vi "Basic Multitone with Amplitudes.vi"(0 "start frequency":dbl=10.0 format="%0.2f", 2 "reset signal":bool, 3 "amplitude":dbl=-1.0 format="%0.2f", 5 "tone amplitudes":dbl[](array[numeric])=[1.0, 2.0] format="%0.2f", 7 "seed":i32=-1, 9 "delta frequency":dbl=100.0 format="%0.2f", 11 "error in (no error)":errorcluster, 12 "sampling info":cluster{"Fs":dbl, "#s":dbl}={"Fs"=1000.0, "#s"=1000.0} {"Fs" format="%.1p"}, 13 "coerce frequencies?":bool, 14 "phase relationship":u16(ring) items=["random", "linear difference", "linear phase"]) -> (4 "signal out":waveform(dbl), 6 "crest factor":dbl format="%0.2f", 10 "actual tone frequencies":dbl[](array[numeric]), 15 "error out":errorcluster)   [LabVIEW 2020, in "NI_MAPro.lvlib"]
doc: "Generates a waveform that is the sum of integer cycle sine tones."
uses:
  NI_MAPro.lvlib
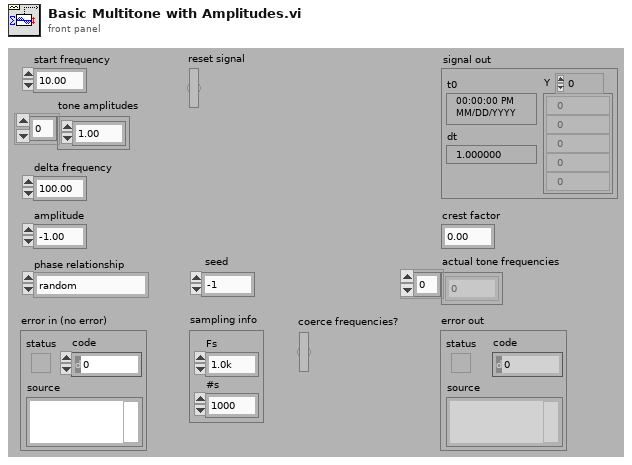
[diagram p1: front panel]
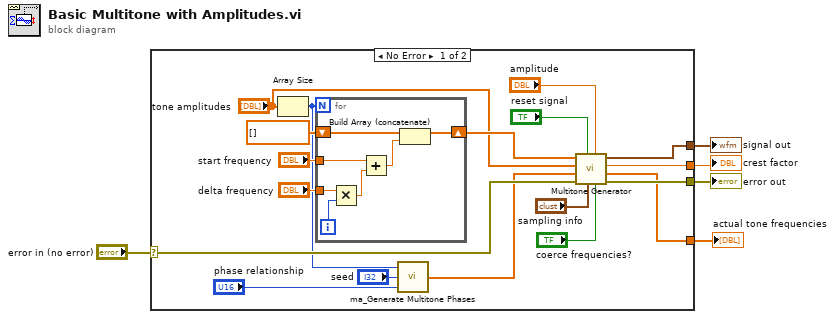
[diagram p0: block diagram]
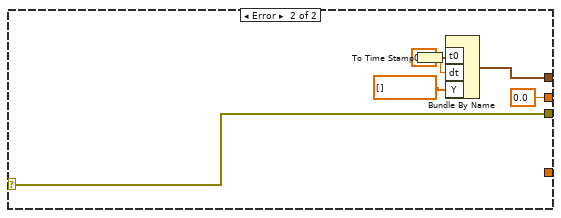
[diagram p2: hidden frame]
diagram:
  n1 = case shown="No Error" "error in (no error)" {
    selector: "error in (no error)" -> [w15 w36]
    tunnel: [w19 w36] -> w5
    tunnel: [w11 0.0 ("crest factor")] -> w3
    tunnel: [w10 w33] -> w2
    tunnel: [w6 _] -> w1
    frame No Error {
      n2 = Array Size(array="tone amplitudes") -> (size(s)=w14:i32)
      n3 = for {
        N: w14 -> [_]
        shift-right: [w29] -> w20
        shift-left: dbl[] [] -> [w30]
        tunnel: "delta frequency" -> [w27]
        tunnel: "start frequency" -> [w26]
        i -> [w28]
        n4 = Multiply(x=w27, y=w28) -> (x*y=w25:dbl)
        n5 = Add(x=w26, y=w25) -> (x+y=w24:dbl)
        n6 = Build Array (concatenate)(w30, w24) -> (w29:dbl[])
      }
      n7 = call "ma_Generate Multitone Phases.vi"("phase relationship"="phase relationship", "seed"="seed", "#tones"=w14) -> ("Tone Phases"=w12:dbl[])
      n8 = call "Multitone Generator.vi"("coerce frequencies?"="coerce frequencies?", "amplitude"="amplitude", "sampling info"="sampling info", "reset signal"="reset signal", "error in (no error)"=w15, "tone phases"=w12, "tone amplitudes"="tone amplitudes", "tone frequencies"=w20) -> ("error out"=w19:errorcluster, "actual tone frequencies"=w6:dbl[], "crest factor"=w11:dbl, "signal out"=w10:waveform(dbl))
    }
    frame Error {
      w35 = 0.0 ("t0")
      n9 = To Time Stamp(1:w35) -> (0:w31:timestamp)
      n10 = Bundle By Name("t0"=w31, "dt"=w35, "Y"=dbl[] []) -> (w33:waveform(dbl))  [unwired: 1 out]
    }
  }
  "error out" <- w5
  "crest factor" <- w3
  "signal out" <- w2
  "actual tone frequencies" <- w1
